vi "AgentAction.vi"(0 "HGF_Visitable":refnum<class "HGF_Visitable.lvclass">, 11 "error in (no error)":errorcluster) -> (4 "dup HGF_Visitable":refnum<class "HGF_Visitable.lvclass">, 15 "error out":errorcluster)   [LabVIEW 2009, in "HGF_VisitorGenerator.lvlib"]
doc: "Placeholder for agents public interface VI"
uses:
  HGF_BaseClasses/HGF_Visitable/HGF_Visitable.lvclass
  HGF_VisitorGenerator.lvlib
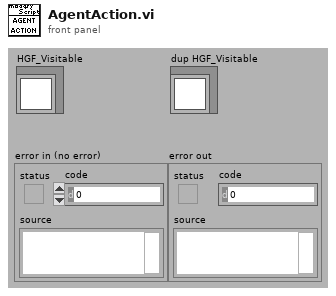
[diagram p1: front panel]
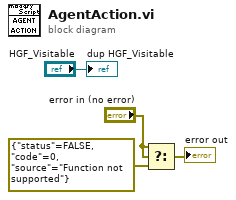
[diagram p0: block diagram]
diagram:
  n1 = Select(t="error in (no error)", s="error in (no error)", f=errorcluster {"status"=FALSE, "code"=0, "source"="Function not supported"} ("error out")) -> (s? t:f=→"error out":errorcluster)
  "dup HGF_Visitable" <- "HGF_Visitable"
